vi "Replace Outside Typedef Const.vi"(6 "Dependent VIs":path[](array[path]), 8 "error in (no error)":errorcluster, 9 "Shared directory":path, 10 "Non-Library VI[]":string[](array[string]), 11 "Measurement Directory":path) -> (0 "error out":errorcluster)   [LabVIEW 2021, in "Multiple Converter.lvlib"]
uses:
  Multiple Converter.lvlib
  <vilib>/Utility/traverseref.llb/TRef TravTarget.ctl
  <vilib>/Utility/traverseref.llb/VI Scripting - Traverse.lvlib
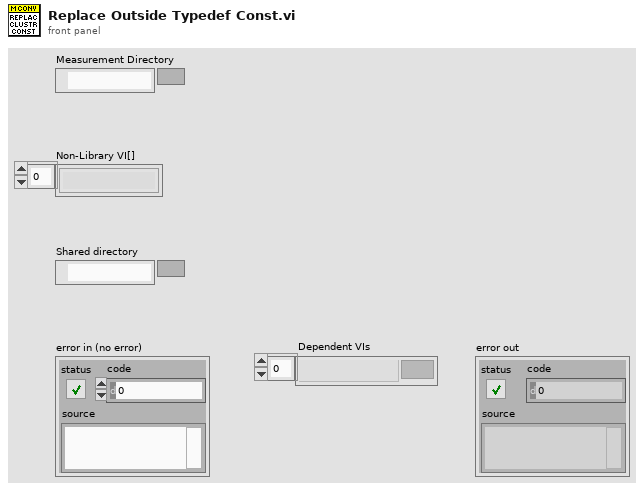
[diagram p1: front panel]
types:
  T1 = typedef "TRef TravTarget.ctl" = enum16{"FP", "BD", "Other"}
  T2 = enum32{"not a typedef", "typedef", "strict typedef", "class private data"}
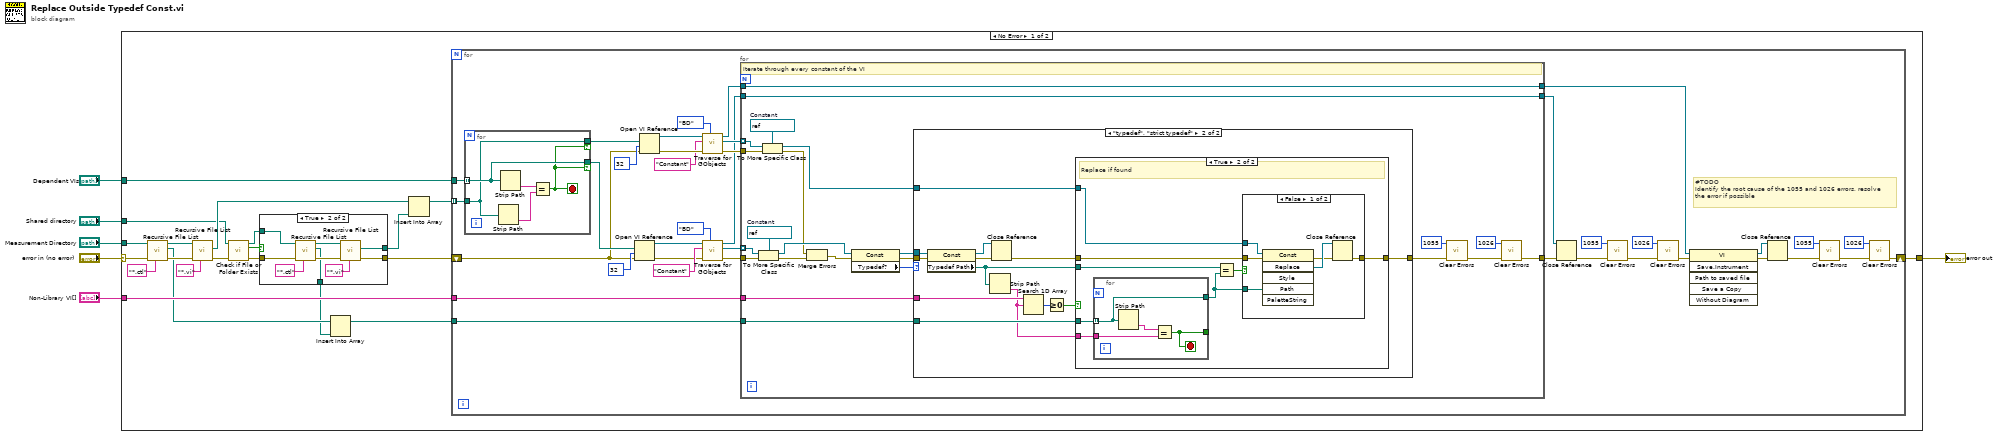
[diagram p0: block diagram]
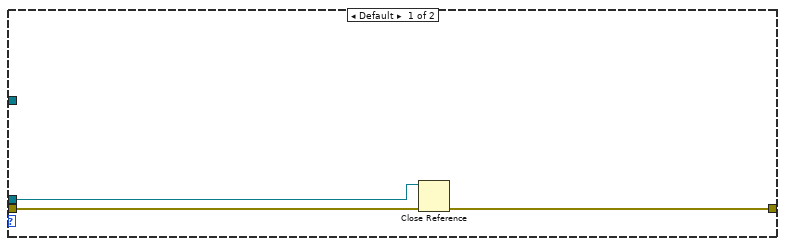
[diagram p2: hidden frame]
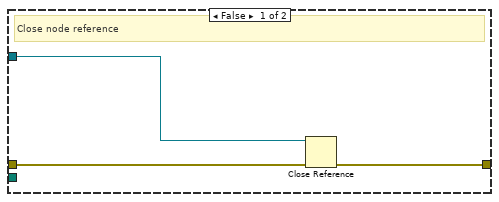
[diagram p3: hidden frame]
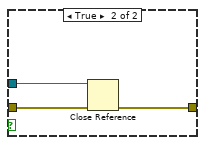
[diagram p4: hidden frame]
diagram:
  n1 = case shown="No Error" "error in (no error)" {
    selector: "error in (no error)" -> [w26 w144]
    tunnel: "Non-Library VI[]" -> [w27 _]
    tunnel: [w24 w144] -> w4
    tunnel: "Measurement Directory" -> [w22 _]
    tunnel: "Shared directory" -> [w8 _]
    tunnel: "Dependent VIs" -> [w7 _]
    frame No Error {
      n2 = call <vilib>:"Recursive File List.vi"("pattern"="*.ctl", "error in (no error)"=w26, "Folder Path"=w22) -> ("error out"=w23:errorcluster, "All Files in Dir"=w19:path[], "dup Folder Path"=w21:path)  [unwired: 4 in, 2 out]
      n3 = call <vilib>:"Recursive File List.vi"("pattern"="*.vi", "error in (no error)"=w23, "Folder Path"=w21) -> ("error out"=w17:errorcluster, "All Files in Dir"=w16:path[])  [unwired: 4 in, 3 out]
      n4 = call <vilib>:"Check if File or Folder Exists.vi"("error in (no error)"=w17, "path"=w8) -> ("error out"=w11:errorcluster, "file or folder exists?"=w10:bool, "dup path"=w9:path)  [unwired: 7 in]
      n5 = case shown="True" w10 {
        tunnel: [w134 w139] -> w18
        tunnel: w11 -> [w134 w138]
        tunnel: [_ w137] -> w13
        tunnel: [_ w136] -> w12
        tunnel: w9 -> [_ w135]
        frame False {
        }
        frame True {
          n6 = call <vilib>:"Recursive File List.vi"("pattern"="*.ctl", "error in (no error)"=w138, "Folder Path"=w135) -> ("error out"=w141:errorcluster, "All Files in Dir"=w137:path[], "dup Folder Path"=w142:path)  [unwired: 4 in, 2 out]
          n7 = call <vilib>:"Recursive File List.vi"("pattern"="*.vi", "error in (no error)"=w141, "Folder Path"=w142) -> ("error out"=w139:errorcluster, "All Files in Dir"=w136:path[])  [unwired: 4 in, 3 out]
        }
      }
      n8 = Insert Into Array(array=w19, new element=w13) -> (w14:path[])  [unwired: 1 in]
      n9 = Insert Into Array(array=w16, new element=w12) -> (w15:path[])  [unwired: 1 in]
      n10 = for {
        tunnel: w14 -> [w64]
        tunnel: w27 -> [w63]
        tunnel: w15 -> [w51] mode=indexing
        shift-right: [w33] -> w24
        shift-left: w18 -> [w44]
        tunnel: w7 -> [w52]
        # "#TODO\nIdentify the root cause of the 1055 and 1026 errors, resolve \nthe error if possible"
        n11 = for {
          tunnel: w52 -> [w131] mode=indexing
          tunnel: w51 -> [w130]
          tunnel: [w131] -> w50 if=w129
          tunnel: [w130] -> w43 if=w129
          stop <- w129 stop-if-true
          n12 = Strip Path(path=w130) -> (name=w132:string)  [unwired: 1 out]
          n13 = Strip Path(path=w131) -> (name=w133:string)  [unwired: 1 out]
          n14 = Equal?(x=w133, y=w132) -> (x = y?=w129:bool)
        }
        n15 = Open VI Reference(vi path=w50, options=32, error in (no error)=w44) -> (vi reference=w56:refnum<vi>, error out=w58:errorcluster)  [unwired: 3 in]
        n16 = Open VI Reference(vi path=w43, options=32, error in (no error)=w44) -> (vi reference=w48:refnum<vi>, error out=w47:errorcluster)  [unwired: 3 in]
        n17 = call <vilib>:"Traverse for GObjects.vi"("Traverse Target"=TRef_TravTarget."BD", "error in (no error)"=w47, "Class Name"="Constant" ("name/order"), "VI Refnum"=w48) -> ("error out"=w42:errorcluster, "References"=w41:refnum<vi>[], "dup VI Refnum"=w40:refnum<vi>)  [unwired: 4 in, 1 out]
        n18 = call <vilib>:"Traverse for GObjects.vi"("Traverse Target"=TRef_TravTarget."BD", "error in (no error)"=w58, "Class Name"="Constant" ("name/order"), "VI Refnum"=w56) -> ("error out"=w62:errorcluster, "References"=w65:refnum<vi>[], "dup VI Refnum"=w39:refnum<vi>)  [unwired: 4 in, 1 out]
        n19 = for {
          tunnel: w65 -> [w88] mode=indexing
          tunnel: w63 -> [w84]
          tunnel: w64 -> [w86]
          tunnel: w42 -> [w81]
          tunnel: w41 -> [w80] mode=indexing
          tunnel: w40 -> [w74]
          tunnel: w39 -> [w75]
          tunnel: [w74] -> w38
          tunnel: [w75] -> w36
          tunnel: w62 -> [w87]
          tunnel: [w67] -> w61
          w82 = refnum<vi> refnum  # Constant
          w85 = refnum<vi> refnum  # Constant
          # "Iterate through every constant of the VI"
          n20 = To More Specific Class(target class=w85, reference=w88, error in=w87) -> (specific class reference=w83:refnum<vi>, error out=w77:errorcluster)
          n21 = To More Specific Class(target class=w82, reference=w80, error in=w81) -> (specific class reference=w79:refnum<vi>, error out=w76:errorcluster)
          n22 = Merge Errors(w76, w77) -> (w78:errorcluster)
          n23 = property class="Const"(reference=w83, error in=w78) -> (reference out=w72:refnum<vi>, error out=w73:errorcluster, "Typedef?"=w71:T2)
          n24 = case shown="\"typedef\", \"strict typedef\"" w71 {
            tunnel: w73 -> [w91 w93]
            tunnel: w72 -> [w89 w99]
            tunnel: [w90 w103] -> w70
            tunnel: w86 -> [_ w101]
            tunnel: w84 -> [_ w100]
            tunnel: w79 -> [_ w94]
            frame Default {
              n25 = Close Reference(reference=w89, error in (no error)=w91) -> (error out=w90:errorcluster)
            }
            frame "typedef", "strict typedef" {
              n26 = property class="Const"(reference=w99, error in=w93) -> (reference out=w95:refnum<vi>, error out=w96:errorcluster, "Typedef Path"=w97:path)
              n27 = Strip Path(path=w97) -> (name=w98:string)  [unwired: 1 out]
              n28 = Close Reference(reference=w95, error in (no error)=w96) -> (error out=w92:errorcluster)
              n29 = Search 1D Array(1D array=w100, element=w98) -> (index of element=w104:i32)  [unwired: 1 in]
              n30 = Greater Or Equal To 0?(x=w104) -> (x >= 0?=w102:bool)
              n31 = case shown="True" w102 {
                tunnel: w92 -> [w107 w115]
                tunnel: [w106 w112] -> w103
                tunnel: w101 -> [_ w114]
                tunnel: w98 -> [_ w113]
                tunnel: w97 -> [_ w111]
                tunnel: w94 -> [w105 w108]
                frame False {
                  # "Close node reference"
                  n32 = Close Reference(reference=w105, error in (no error)=w107) -> (error out=w106:errorcluster)
                }
                frame True {
                  # "Replace if found"
                  n33 = for {
                    tunnel: w114 -> [w126] mode=indexing
                    tunnel: w113 -> [w127]
                    tunnel: [w126] -> w110
                    tunnel: [w125] -> _
                    stop <- w125 stop-if-true
                    n34 = Strip Path(path=w126) -> (name=w128:string)  [unwired: 1 out]
                    n35 = Equal?(x=w128, y=w127) -> (x = y?=w125:bool)
                  }
                  n36 = Equal?(x=w111, y=w110) -> (x = y?=w109:bool)
                  n37 = case shown="False" w109 {
                    tunnel: w115 -> [w121 w124]
                    tunnel: [w119 w123] -> w112
                    tunnel: w110 -> [w118 _]
                    tunnel: w108 -> [w116 w122]
                    frame False {
                      n38 = invoke class="Const" method="Replace"(reference=w116, error in=w121, "Path"=w118) -> (error out=w117:errorcluster, "Replace"=w120:refnum<vi>)  [unwired: 3 in, 4 out]
                      n39 = Close Reference(reference=w120, error in (no error)=w117) -> (error out=w119:errorcluster)
                    }
                    frame True {
                      n40 = Close Reference(reference=w122, error in (no error)=w124) -> (error out=w123:errorcluster)
                    }
                  }
                }
              }
            }
          }
          n41 = call <vilib>:"Clear Errors.vi"("error in (no error)"=w70, "specific error code to clear (0: all)"=1055) -> ("error out"=w69:errorcluster)  [unwired: 4 in, 1 out]
          n42 = call <vilib>:"Clear Errors.vi"("error in (no error)"=w69, "specific error code to clear (0: all)"=1026) -> ("error out"=w67:errorcluster)  [unwired: 4 in, 1 out]
        }
        n43 = Close Reference(reference=w36, error in (no error)=w61) -> (error out=w37:errorcluster)
        n44 = call <vilib>:"Clear Errors.vi"("error in (no error)"=w37, "specific error code to clear (0: all)"=1055) -> ("error out"=w31:errorcluster)  [unwired: 4 in, 1 out]
        n45 = call <vilib>:"Clear Errors.vi"("error in (no error)"=w31, "specific error code to clear (0: all)"=1026) -> ("error out"=w35:errorcluster)  [unwired: 4 in, 1 out]
        n46 = invoke class="VI" method="Save.Instrument"(reference=w38, error in=w35) -> (reference out=w54:refnum<vi>, error out=w55:errorcluster)  [unwired: 4 in, 4 out]
        n47 = Close Reference(reference=w54, error in (no error)=w55) -> (error out=w57:errorcluster)
        n48 = call <vilib>:"Clear Errors.vi"("error in (no error)"=w57, "specific error code to clear (0: all)"=1055) -> ("error out"=w29:errorcluster)  [unwired: 4 in, 1 out]
        n49 = call <vilib>:"Clear Errors.vi"("error in (no error)"=w29, "specific error code to clear (0: all)"=1026) -> ("error out"=w33:errorcluster)  [unwired: 4 in, 1 out]
      }
    }
    frame Error {
    }
  }
  "error out" <- w4
